vi "Get Tag Value_ByRef.vi"(8 "error in (no error)":errorcluster, 10 "Tag Ref in":refnum<data-value>) -> (0 "error out":errorcluster, 1 "Value":variant, 2 "Tag Ref out":refnum<data-value>, 5 "Timestamp":timestamp)   [LabVIEW 2020, in "Tag Engine.lvlib" / "Tag Core.lvclass"]
doc: "_SubVI_"
uses:
  Tag Core.lvclass
  Tag/Tag.lvclass
  Tag/Tag.lvclass/Tag.ctl
  Tag Core.lvclass/Tag Core.ctl
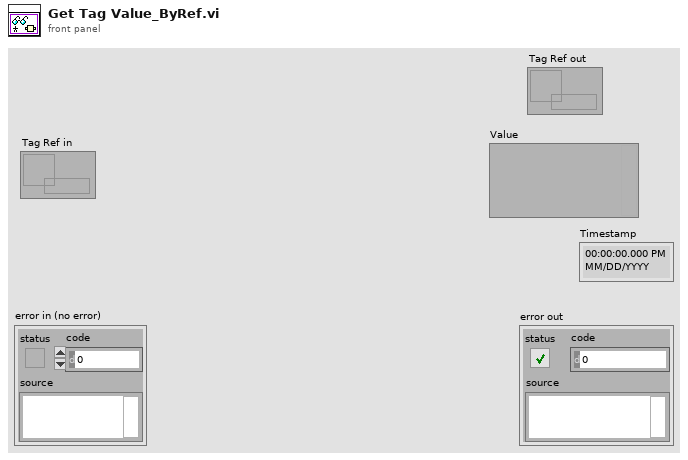
[diagram p1: front panel]
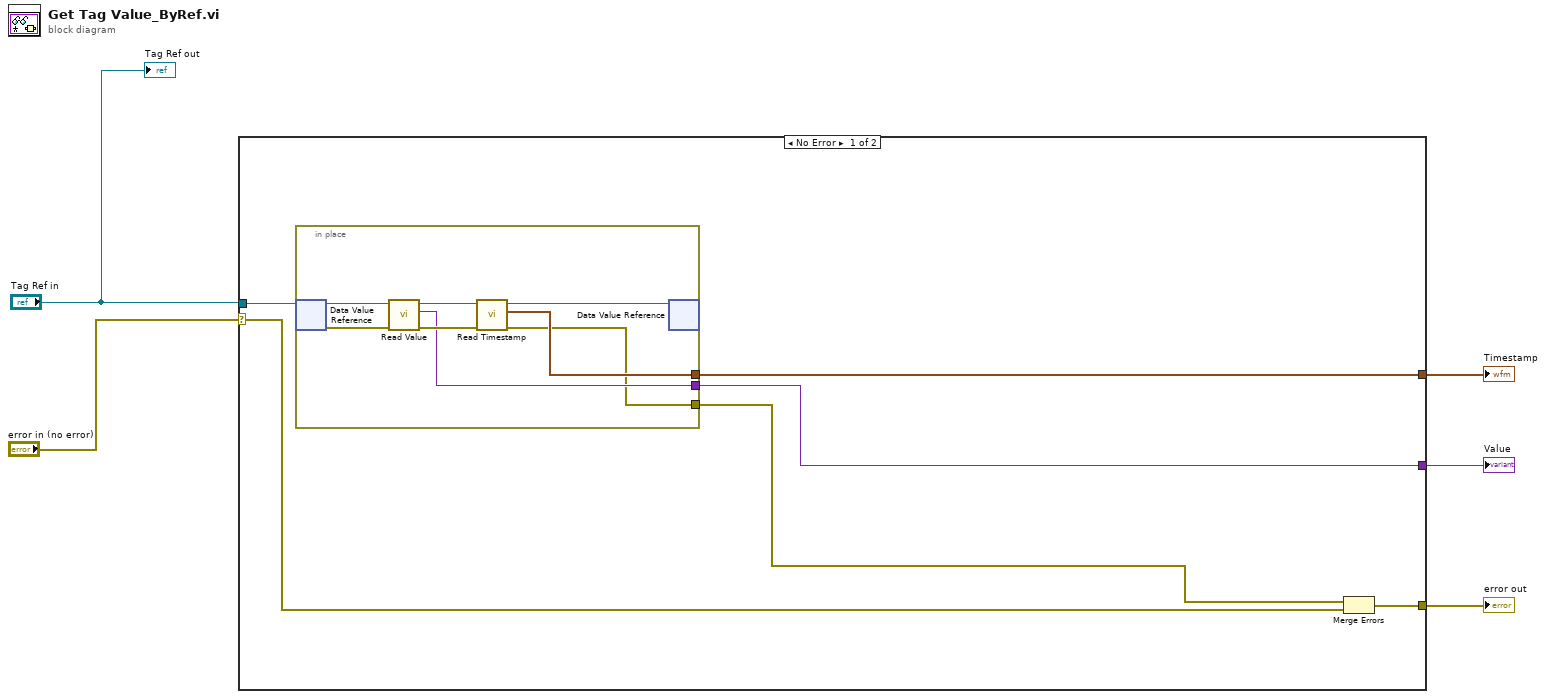
[diagram p0: block diagram]
diagram:
  n1 = case shown="No Error" "error in (no error)" {
    selector: "error in (no error)" -> [w9 w20]
    tunnel: "Tag Ref in" -> [w11 _]
    tunnel: [w10 _] -> w3
    tunnel: [w6 _] -> w4
    tunnel: [w8 w20] -> w5
    frame No Error {
      n2 = in-place {
        in-place-border: [w15] -> w6
        in-place-border: [w14] -> w10
        in-place-border: [w13] -> w7
        n3 = in-place-dvr #1(w11) -> (w19:refnum<class "Tag.lvclass">, w18:errorcluster)
        n4 = call "Read Value.vi"("error in (no error)"=w18, "Tag in"=w19) -> ("error out"=w16:errorcluster, "Value"=w15:variant, "Tag out"=w17:refnum<class "Tag.lvclass">)  [unwired: 7 in]
        n5 = call "Read Timestamp.vi"("error in (no error)"=w16, "Tag in"=w17) -> ("error out"=w13:errorcluster, "Timestamp"=w14:timestamp, "Tag out"=w12:refnum<class "Tag.lvclass">)  [unwired: 7 in]
        n6 = in-place-dvr #1(w12) -> ()  [unwired: 2 out]
      }
      n7 = Merge Errors(w7, w9) -> (w8:errorcluster)
    }
    frame Error {
    }
  }
  "error out" <- w5
  "Value" <- w4
  "Timestamp" <- w3
  "Tag Ref out" <- "Tag Ref in"
